vi "Close Account.vi"(8 "错误输入":errorcluster, 11 "帐户信息":T1) -> (0 "错误输出":errorcluster)   [LabVIEW 2012]
uses:
  Account Info.ctl
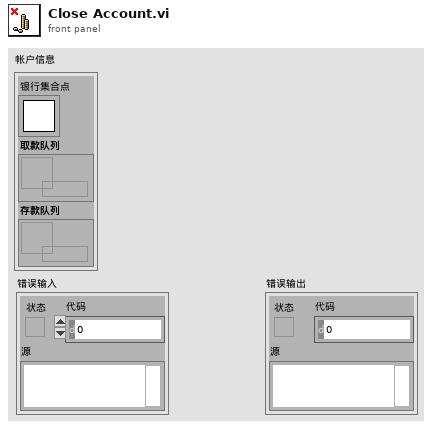
[diagram p1: front panel]
types:
  T1 = typedef "Account Info.ctl" = cluster{"银行集合点":T2, "取款队列":refnum<queue>, "存款队列":refnum<queue>}
  T2 = typedef "Rendezvous RefNum" = refnum<k1>
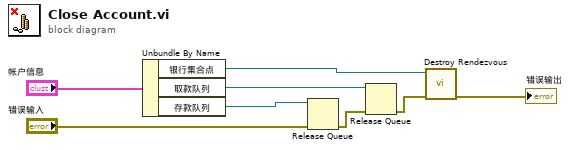
[diagram p0: block diagram]
diagram:
  n1 = Unbundle By Name ("按名称解除捆绑")("帐户信息") -> ("银行集合点"=w7:T2, "取款队列"=w4:refnum<queue>, "存款队列"=w6:refnum<queue>)
  n2 = Release Queue ("释放队列引用")(queue=w6, error in (no error)="错误输入") -> (error out=w5:errorcluster)  [unwired: 1 in, 2 out]
  n3 = Release Queue ("释放队列引用")(queue=w4, error in (no error)=w5) -> (error out=w3:errorcluster)  [unwired: 1 in, 2 out]
  n4 = call <vilib>:"Destroy Rendezvous.vi"("error in (no error)"=w3, "rendezvous"=w7) -> ("error out"=→"错误输出":errorcluster)  [unwired: 4 in, 1 out]
